vi "B&K 9120 series control panel.vi"() -> ()   [LabVIEW 2014]
uses:
  Serial_Config.ctl
  Meter_VI.ctl
  B&K Precision 9120 series.lvclass
  <vilib>/Utility/error.llb/DialogType.ctl
panel:
  out "Enabled":bool
  in  "Output Enable":bool
  in  "Limit Setpoint":T1={"Voltage"=1.0, "Current"=1.0} caption="Measured" {"Current" scale=0.0..1.2 scale format="%#_5f"; "Voltage" scale=0.0..72.0 scale format="%#_5f"}
  out "Measured":T1 {"Current" scale=0.0..1.2 scale format="%#_5f"; "Voltage" scale=0.0..72.0 scale format="%#_5f"}
  in  "stop":bool
  out "Error Status":errorcluster
  in  "Connection":T3={"Serial Config"={"Baud"=9600, "Flow Ctl"=0, "Parity"=0}, "VISA resource name"="COM1", "Connect"=FALSE, "Status"="", "Connected"=FALSE} {"Serial Config"."Parity" items=["None", "Odd", "Even"]; "Serial Config"."Flow Ctl" items=["None"]; "Serial Config"."Baud" items=["4800"=4800, "9600"=9600, "19200"=19200, "38400"=38400]}
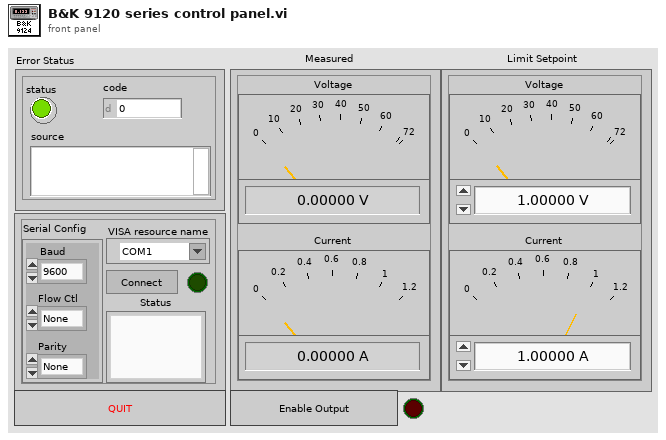
[diagram p1: front panel]
types:
  T1 = typedef "Meter_VI.ctl" = cluster{"Voltage":dbl, "Current":dbl}
  T2 = typedef "B&K Precision 9120 series.lvclass/Serial_Config.ctl" = cluster{"Baud":u32, "Flow Ctl":u16, "Parity":u16}
  T3 = cluster{"Serial Config":T2, "VISA resource name":refnum<visa-resource-name>, "Connect":bool, "Status":string, "Connected":bool}
  T4 = typedef "DialogType.ctl" = u16
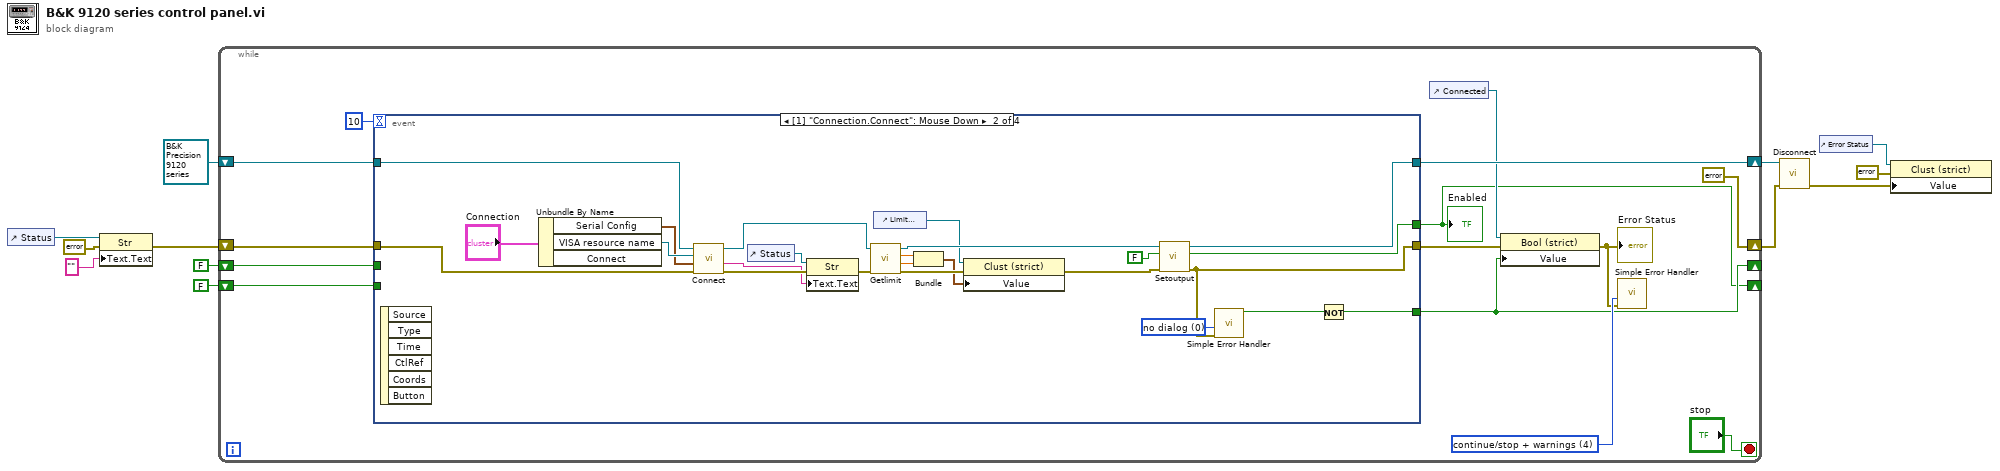
[diagram p0: block diagram]
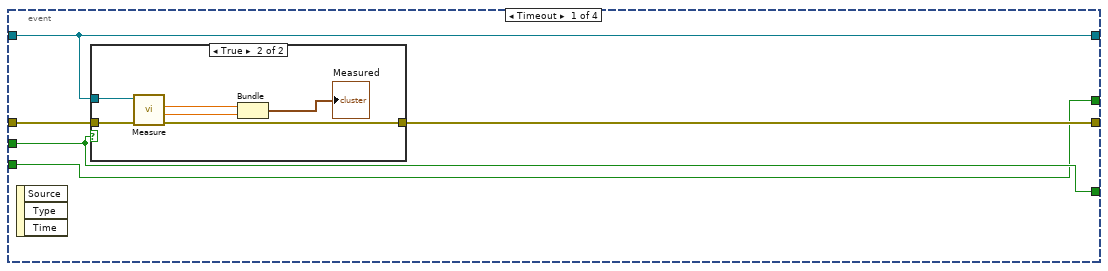
[diagram p2: hidden frame]
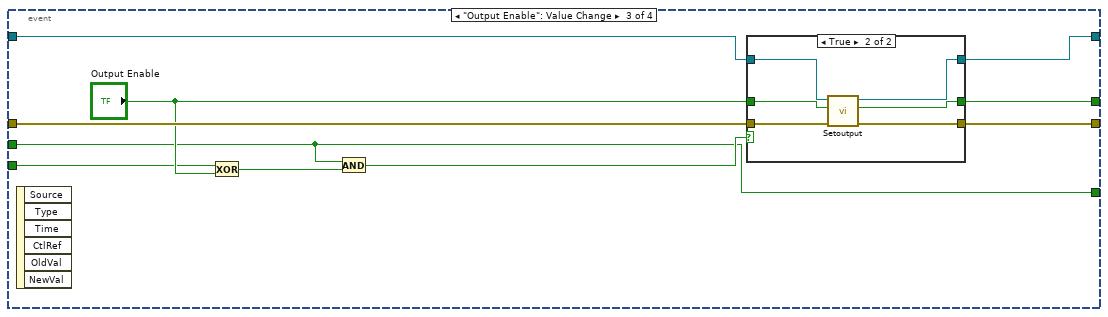
[diagram p4: hidden frame]
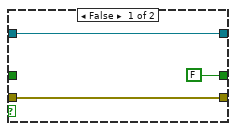
[diagram p5: hidden frame]
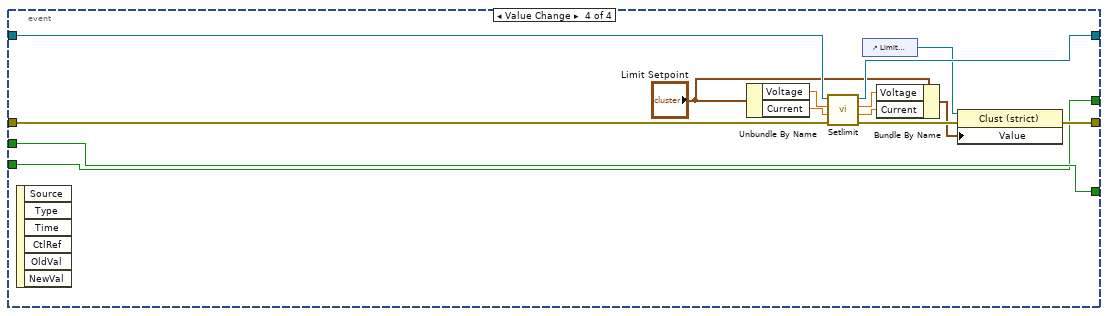
[diagram p6: hidden frame]
diagram:
  n1 = control-ref of="Status"() -> (w6:refnum<vi>)
  n2 = property class="Str"(reference=w6, error in=errorcluster {"status"=FALSE, "code"=0, "source"=""} ("error in (no error)"), "Text.Text"="") -> (error out=w3:errorcluster)  [unwired: 1 out]
  n3 = while {
    shift-right: [errorcluster {"status"=FALSE, "code"=0, "source"=""} ("error out")] -> w10
    shift-left: w3 -> [w26]
    shift-right: [w25] -> w11
    shift-left: refnum<class "B&K Precision 9120 series.lvclass"> refnum ("B&K Precision 9120 series.lvclass") -> [w24]
    shift-right: [w16] -> _
    shift-left: FALSE -> [w19]
    shift-right: [w13] -> _
    shift-left: FALSE ("actual_state") -> [w15]
    stop <- "stop" stop-if-true
    w21 = T4 4 items=["no dialog", "OK message", "continue or stop message", "OK message + warnings", "continue/stop + warnings"] ("type of dialog (OK msg:1)")
    n4 = event shown="[1] \"Connection.Connect\": Mouse Down" {
      selector: _ -> [_ _ _ _]
      dyn-events: _ -> [_ _ _ _]
      timeout: 10 -> [_ _ _ _]
      tunnel: w24 -> [w28 w62 w72 w95]
      tunnel: w26 -> [w31 w59 w69 w91]
      tunnel: [w30 w40 w68 w84] -> w17
      tunnel: [w28 w44 w70 w94] -> w25
      tunnel: w19 -> [w29 _ w63 w83]
      tunnel: [w29 w54 w63 w83] -> w16
      tunnel: [w27 w41 w71 w82] -> w13
      tunnel: w15 -> [w27 _ w66 w82]
      event Timeout {
        n5 = event-data() -> ()  [unwired: 1 in, 3 out]
        n6 = case shown="True" w29 {
          tunnel: w28 -> [_ w38]
          tunnel: w31 -> [w32 w37]
          tunnel: [w32 w36] -> w30
          frame False {
          }
          frame True {
            n7 = call "Measure.vi"("error in (no error)"=w37, "B&K Precision 9120 series in"=w38) -> ("error out"=w36:errorcluster, "Current"=w34:dbl, "Voltage"=w35:dbl)  [unwired: 6 in, 1 out]
            n8 = Bundle("Voltage"=w35, "Current"=w34) -> (→"Measured":cluster{"Voltage":dbl, "Current":dbl})  [unwired: 1 in]
          }
        }
      }
      event "Connection.Connect": Mouse Down {
        w39 = T4 0 items=["no dialog", "OK message", "continue or stop message", "OK message + warnings", "continue/stop + warnings"] ("type of dialog (OK msg:1)")
        n9 = event-data() -> ()  [unwired: 1 in, 6 out]
        n10 = Unbundle By Name("Connection") -> ("Serial Config"=w60:T2, "VISA resource name"=w61:refnum<visa-resource-name>)  [unwired: 1 out]
        n11 = call "Connect.vi"("error in (no error)"=w59, "Serial Config"=w60, "VISA resource name"=w61, "B&K Precision 9120 series in"=w62) -> ("error out"=w57:errorcluster, "result"=w56:string, "B&K Precision 9120 series out"=w52:refnum<class "B&K Precision 9120 series.lvclass">)  [unwired: 5 in]
        n12 = control-ref of="Status"() -> (w58:refnum<vi>)
        n13 = property class="Str"(reference=w58, error in=w57, "Text.Text"=w56) -> (error out=w50:errorcluster)  [unwired: 1 out]
        n14 = call "Getlimit.vi"("error in (no error)"=w50, "B&K Precision 9120 series in"=w52) -> ("error out"=w47:errorcluster, "Current read"=w48:dbl, "Voltage read"=w49:dbl, "B&K Precision 9120 series out"=w51:refnum<class "B&K Precision 9120 series.lvclass">)  [unwired: 6 in]
        n15 = control-ref of="Limit Setpoint"() -> (w46:refnum<vi>)
        n16 = Bundle("Voltage read"=w49, "Current read"=w48) -> (w45:cluster{"Voltage read":dbl, "Current read":dbl})  [unwired: 1 in]
        n17 = property class="Clust (strict)"(reference=w46, error in=w47, "Value"=w45) -> (error out=w43:errorcluster)  [unwired: 1 out]
        n18 = call "Setoutput.vi"("error in (no error)"=w43, "enable"=FALSE, "B&K Precision 9120 series in"=w51) -> ("error out"=w40:errorcluster, "actual_state"=w41:bool, "B&K Precision 9120 series out"=w44:refnum<class "B&K Precision 9120 series.lvclass">)  [unwired: 6 in]
        n19 = call <vilib>:"Simple Error Handler.vi"("type of dialog (OK msg:1)"=w39, "error in (no error)"=w40) -> ("error?"=w53:bool)  [unwired: 3 in, 4 out]
        n20 = Not(x=w53) -> (.not. x?=w54:bool)
      }
      event "Output Enable": Value Change {
        n21 = event-data() -> ()  [unwired: 1 in, 6 out]
        n22 = Exclusive Or(1:"Output Enable", 2:w66) -> (0:w65:bool)
        n23 = And(x=w63, y=w65) -> (x .and. y?=w64:bool)
        n24 = case shown="True" w64 {
          tunnel: w72 -> [w75 w81]
          tunnel: [FALSE ("actual_state") w80] -> w71
          tunnel: [w75 w79] -> w70
          tunnel: w69 -> [w73 w78]
          tunnel: [w73 w77] -> w68
          tunnel: "Output Enable" -> [_ w76]
          frame False {
          }
          frame True {
            n25 = call "Setoutput.vi"("error in (no error)"=w78, "enable"=w76, "B&K Precision 9120 series in"=w81) -> ("error out"=w77:errorcluster, "actual_state"=w80:bool, "B&K Precision 9120 series out"=w79:refnum<class "B&K Precision 9120 series.lvclass">)  [unwired: 6 in]
          }
        }
      }
      event Value Change {
        n26 = event-data() -> ()  [unwired: 1 in, 6 out]
        n27 = Unbundle By Name("Limit Setpoint") -> ("Voltage"=w93:dbl, "Current"=w92:dbl)
        n28 = call "Setlimit.vi"("error in (no error)"=w91, "Current"=w92, "Voltage"=w93, "B&K Precision 9120 series in"=w95) -> ("error out"=w89:errorcluster, "Current read"=w86:dbl, "Voltage read"=w87:dbl, "B&K Precision 9120 series out"=w94:refnum<class "B&K Precision 9120 series.lvclass">)  [unwired: 4 in]
        n29 = control-ref of="Limit Setpoint"() -> (w90:refnum<vi>)
        n30 = Bundle By Name(cluster="Limit Setpoint", "Voltage"=w87, "Current"=w86) -> (w85:T1)
        n31 = property class="Clust (strict)"(reference=w90, error in=w89, "Value"=w85) -> (error out=w84:errorcluster)  [unwired: 1 out]
      }
    }
    "Enabled" <- w13
    n32 = control-ref of="Connected"() -> (w18:refnum<vi>)
    n33 = property class="Bool (strict)"(reference=w18, error in=w17, "Value"=w16) -> (error out=w14:errorcluster)  [unwired: 1 out]
    "Error Status" <- w14
    n34 = call <vilib>:"Simple Error Handler.vi"("type of dialog (OK msg:1)"=w21, "error in (no error)"=w14) -> ()  [unwired: 3 in, 5 out]
  }
  n35 = call "Disconnect.vi"("error in (no error)"=w10, "B&K Precision 9120 series in"=w11) -> ("error out"=w8:errorcluster)  [unwired: 9 in]
  n36 = control-ref of="Error Status"() -> (w9:refnum<vi>)
  n37 = property class="Clust (strict)"(reference=w9, error in=errorcluster {"status"=FALSE, "code"=0, "source"=""} ("error in (no error)"), "Value"=w8) -> ()  [unwired: 2 out]
